vi "MM with MFC Challenge.vi"(8 "error in":errorcluster, 11 "objects IN":T1) -> (0 "error out":errorcluster, 3 "objects OUT":T1)   [LabVIEW 2011]
uses:
  Controls/Class Objects.ctl
  Modules/File/Configuration/Configuration.lvclass
  Modules/Hardware/PID/PID.lvclass
  Modules/Hardware/Power Supply/Power Supply.lvclass
  Modules/Hardware/Mass Flow Controller/Mass Flow Controller.lvclass
  Modules/Hardware/Valve Controller/Valve Controller.lvclass
  Modules/Hardware/Multimeter/Multimeter.lvclass
  Modules/Hardware/Vapour Generator/Vapour Generator.lvclass
  Modules/File/TDMS/TDMS.lvclass
  Controls/User Interface Action.ctl
  Functional Global Data/Device Params Global.ctl
  Modules/File/TDMS/Data Type.ctl
  Controls/TDMS File Handling.ctl
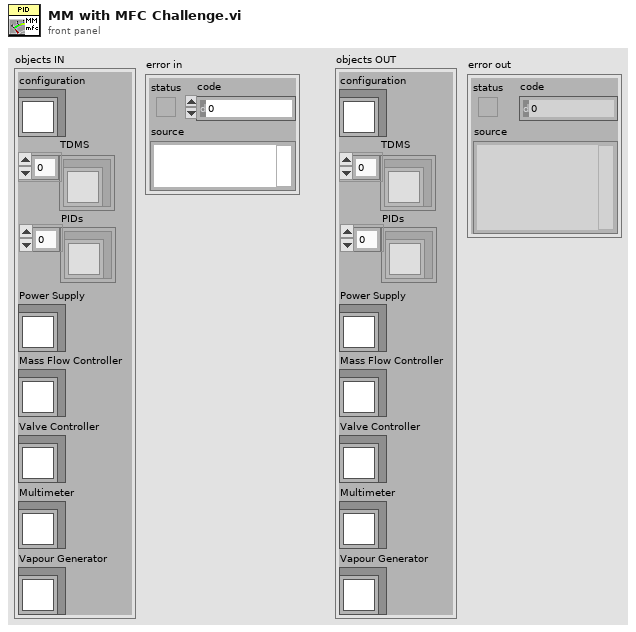
[diagram p1: front panel]
types:
  T1 = typedef "Class Objects.ctl" = cluster{"configuration":refnum<class "Configuration.lvclass">, "TDMS":refnum<class "TDMS.lvclass">[], "Power Supply":refnum<class "Power Supply.lvclass">, "Mass Flow Controller":refnum<class "Mass Flow Controller.lvclass">, "Valve Controller":refnum<class "Valve Controller.lvclass">, "Multimeter":refnum<class "Multimeter.lvclass">, "Vapour Generator":refnum<class "Vapour Generator.lvclass">, "PIDs":refnum<class "PID.lvclass">[]}
  T2 = typedef "User Interface Action.ctl" = enum16{"Initialize", "Data Acquisition Disable", "Data View Disable", "Sample Set", "Sample Set 2D Data", "Sample Set x0 & dx", "Sample Add", "Sample Set Cursor", "Sample Set Offset & Multiplier", "Sample Set Axis Labels", "Sample Parameters Disabled", "Sample Parameters Update", "Run Update", "Run Set Offset & Multiplier", "Run Set Axis Labels", "Run Set Cursor", "Run Set Disabled", "Run Parameters Update", "Run Parameters Disabled", "Run Number Set", "Run Number Set Range", "Run Number Set Disabled", "Sample Number Set", "Sample Number Set Range", "Notes Set Value", "Update Plot", "Set Plot Parameters", "Update Concentration Plot", "Time Set", "Clear DAQ Display", "Clear Analysis Display", "Status Bar Set", "Progress Bar Set", "Display Mode Set", "Experiment Type Set", "Analysis Plot Average Set", "Stop"}
  T3 = typedef "Device Params Global.ctl" = enum16{"Initialize", "Get Device Settings", "Get Device Connections", "Set Device Settings", "Set Device Connections", "Get All Device Properties"}
  T4 = typedef "TDMS.lvclass/Data Type.ctl" = enum16{"I16", "Double", "Waveform"}
  T5 = typedef "TDMS File Handling.ctl" = enum16{"Add TDMS File", "Get Active TDMS File", "Set Active TDMS File", "Set Active TDMS File Index"}
  T6 = typedef "Device Settings.ctl" = cluster{"PID":cluster{"B-M PID":T7, "INL PID":T8}, "Power Supply":cluster{"Source Value":dbl, "Source Value Units":T9, "Source Mode":T10, "Limits":T11, "Output":bool}, "Mass Flow Controller":cluster{"MFC Flow Rate":dbl, "MFC Valve Status":T14}, "Valve Controller":cluster{"Valve Assembly":T15}, "Multimeter":cluster{"Agilent 3458A":cluster{"Measurement Configuration":T17, "Measurement Integration":T18}}, "Vapour Generator":cluster{"Owlstone Permeation Tube":T19, "Owlstone GEN-SYS Setpoints":T21}}
  T7 = typedef "Baseline Mocon piD-Tech plus.lvclass/Settings.ctl" = cluster{"Detector Sampling Frequency":dbl}
  T8 = typedef "INL PID.lvclass/Settings.ctl" = cluster{"Sampling Frequency":dbl, "Integration Time":dbl, "Integration Periods":u8, "Grid Voltage":dbl}
  T9 = typedef "Power Supply.lvclass/Source Units.ctl" = enum16{"volts", "millivolts", "microvolts", "amps", "milliamps", "microamps", "nanoamps"}
  T10 = typedef "Power Supply.lvclass/Source Mode.ctl" = enum16{"Volts", "Current"}
  T11 = typedef "Power Supply.lvclass/Protection Limits.ctl" = cluster{"Voltage Limit":dbl, "Voltage Limit Units":T12, "Current Limit":dbl, "Current Limit Units":T13, "Voltage Trip/Cmpl":dbl, "Voltage Trip/Cmpl Units":T12, "Current Trip/Cmpl":dbl, "Current Trip/Cmpl Units":T13}
  T12 = typedef "Power Supply.lvclass/Voltage Units.ctl" = enum16{"volts", "millivolts", "microvolts"}
  T13 = typedef "Power Supply.lvclass/Current Units.ctl" = enum16{"amps", "milliamps", "microamps", "nanoamps"}
  T14 = typedef "Mass Flow Controller.lvclass/Valve Status.ctl" = enum16{"Open", "Closed"}
  T15 = typedef "Valve Controller.lvclass/Valve Assembly.ctl" = cluster{"Valve 1":T16, "Valve 2":T16, "Valve 3":T16, "Valve 4":T16, "Valve 5":T16}
  T16 = typedef "Valve Controller.lvclass/Status.ctl" = u16
  T17 = typedef "Agilent 3458A.lvclass/Measurement Configuration.ctl" = cluster{"Function":enum16{"DC Voltage", "AC Voltage", "AC + DC Voltage", "DC Current", "AC Current", "AC + DC Current", "2-Wire Resistance", "4-Wire Resistance", "Frequency", "Period", "Direct Sampling DC", "Direct Sampling AC", "Sub-Sampling DC", "Sub-Sampling AC"}, " Manual Resolution":enum16{"4.5", "5.5", "6.5", "7.5", "8.5"}, "Frequency Source":enum16{"AC + DC Current", "AC + DC Voltage", "AC Current", "AC Voltage"}, "Auto Range":enum16{"OFF", "ON", "ONCE"}}
  T18 = typedef "Agilent 3458A.lvclass/Measurement Integration.ctl" = cluster{"Power Line Cycles":dbl}
  T19 = typedef "Owlstone GEN-SYS.lvclass/Permeation Tube.ctl" = cluster{"Tube":T20, "Molecular Weight":dbl, "Calibration Temperature\n(Celcius)":i32, "Permeation Rate \n(ng/min)":i32}
  T20 = typedef "Owlstone GEN-SYS.lvclass/Permeation Tube Gas.ctl" = enum16{"Isobutylene 27 Nov 2012", "Ammonia 29 Sep 2012", "DMMP Tube A 3 July 2014", "DMMP Tube B 3 July 2014"}
  T21 = typedef "Owlstone GEN-SYS.lvclass/Gen-Sys Setpoints.ctl" = cluster{"OVG-4":cluster{"Oven Temperature":i32, "Sample Flow Rate":i32, "Split Flow Status":u16, "Split Flow Rate":i32}, "OHG-4":cluster{"Wet Air Flow":i32}}
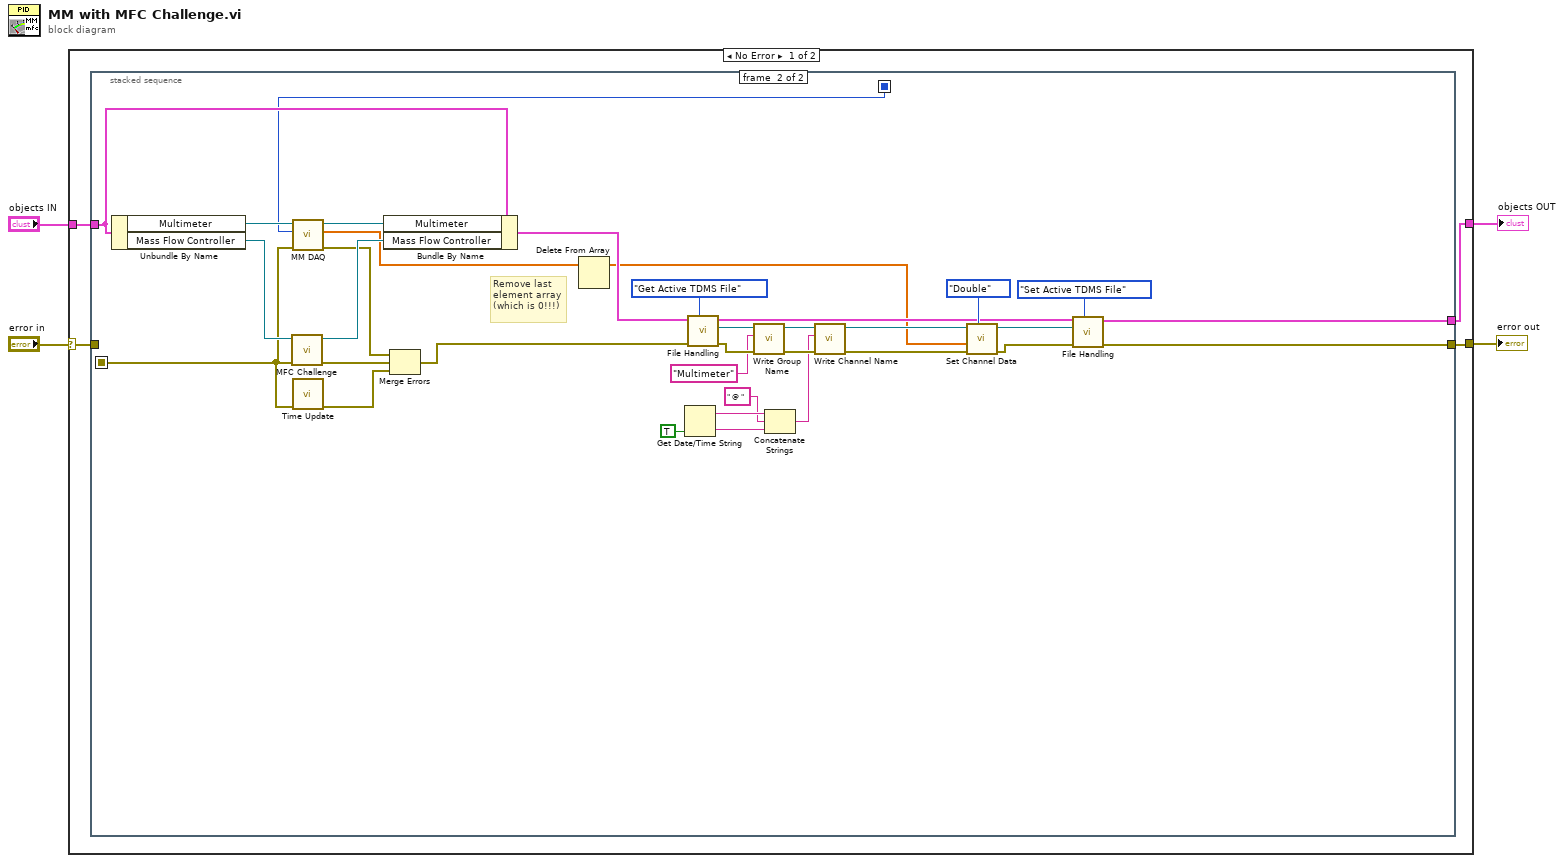
[diagram p0: block diagram]
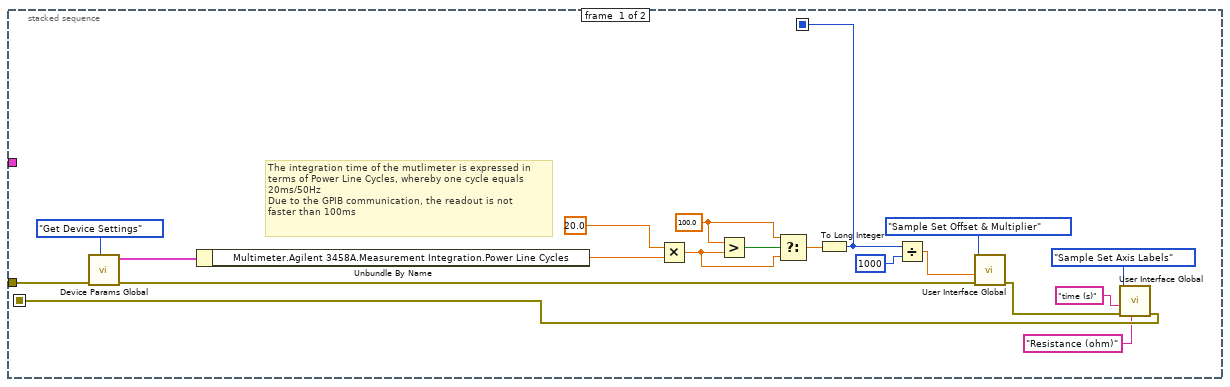
[diagram p2: hidden frame]
diagram:
  n1 = case shown="No Error" "error in" {
    selector: "error in" -> [w5 w62]
    tunnel: "objects IN" -> [w8 w63]
    tunnel: [w6 w63] -> w3
    tunnel: [w7 w62] -> w1
    frame No Error {
      n2 = stacked-sequence {
        seq-local: [w16 _] -> [_ w36]
        seq-local: [w10 _] -> [_ w29]
        tunnel: w8 -> [_ w61]
        tunnel: [_ w30] -> w7
        tunnel: [_ w53] -> w6
        tunnel: w5 -> [w25 _]
        frame #0 {
          w21 = 100.0 ("x")
          # "The integration time of the mutlimeter is expressed in\nterms of Power Line Cycles, whereby one cycle equals\n20ms/50Hz\nDue to the GPIB communication, the readout is not\nfaster than 100ms"
          n3 = call "Device Params Global.vi"("action"=Device_Params_Global."Get Device Settings", "error in"=w25) -> ("error out"=w17:errorcluster, "Device Settings OUT"=w26:T6)  [unwired: 7 in, 1 out]
          n4 = Unbundle By Name(w26) -> ("Multimeter.Agilent 3458A.Measurement Integration.Power Line Cycles"=w24:dbl)
          n5 = Multiply(x=20.0, y=w24) -> (x*y=w20:dbl)
          n6 = Greater?(x=w21, y=w20) -> (0:w22:bool)
          n7 = Select(t=w21, s=w22, f=w20) -> (s? t:f=w19:dbl)
          n8 = To Long Integer(number=w19) -> (32bit integer=w16:i32)
          n9 = Divide(x=w16, y=1000) -> (x/y=w14:dbl)
          n10 = call "User Interface Global.vi"("error in"=w17, "data1"=w14, "action"=User_Interface_Action."Sample Set Offset & Multiplier") -> ("error out"=w12:errorcluster)  [unwired: 8 in]
          n11 = call "User Interface Global.vi"("data2"="Resistance (ohm)", "error in"=w12, "data1"="time (s)", "action"=User_Interface_Action."Sample Set Axis Labels") -> ("error out"=w10:errorcluster)  [unwired: 7 in]
        }
        frame #1 {
          # "Remove last\nelement array\n(which is 0!!!)"
          n12 = Unbundle By Name(w61) -> ("Multimeter"=w38:refnum<class "Multimeter.lvclass">, "Mass Flow Controller"=w40:refnum<class "Mass Flow Controller.lvclass">)
          n13 = call "MFC Challenge.vi"("error in"=w29, "Mass Flow Controller in"=w40) -> ("error out"=w34:errorcluster, "Mass Flow Controller out"=w39:refnum<class "Mass Flow Controller.lvclass">)  [unwired: 8 in]
          n14 = call "MM DAQ.vi"("error in"=w29, "DAQ dt"=w36, "Multimeter in"=w38) -> ("error out"=w35:errorcluster, "Data"=w32:dbl[], "Multimeter out"=w37:refnum<class "Multimeter.lvclass">)  [unwired: 6 in]
          n15 = call "Time Update.vi"("error in"=w29) -> ("error out"=w28:errorcluster)  [unwired: 10 in]
          n16 = Bundle By Name(cluster=w61, "Multimeter"=w37, "Mass Flow Controller"=w39) -> (w59:T1)
          n17 = Merge Errors(w35, w34, w28) -> (w33:errorcluster)
          n18 = Delete From Array(array=w32) -> (array with subset deleted=w31:dbl[])  [unwired: 2 in, 1 out]
          n19 = Get Date/Time String(want seconds? (F)=TRUE) -> (date string=w49:string, time string=w44:string)  [unwired: 2 in]
          n20 = call "File Handling.vi"("TDMS File Handling"=TDMS_File_Handling."Get Active TDMS File", "error in"=w33, "Class objects"=w59) -> ("error out"=w51:errorcluster, "TDMS File"=w52:refnum<class "TDMS.lvclass">, "Class objects"=w54:T1)  [unwired: 6 in]
          n21 = call-dynamic "Write Group Name.vi"("error in (no error)"=w51, "Group Name"="Multimeter", "TDMS in"=w52) -> ("error out"=w47:errorcluster, "TDMS out"=w48:refnum<class "TDMS.lvclass">)  [unwired: 7 in]
          n22 = Concatenate Strings(w49, " @ " ("string"), w44) -> (w42:string)
          n23 = call-dynamic "Write Channel Name.vi"("error in (no error)"=w47, "Channel Name"=w42, "TDMS in"=w48) -> ("error out"=w46:errorcluster, "TDMS out"=w45:refnum<class "TDMS.lvclass">)  [unwired: 7 in]
          n24 = call-dynamic "Set Channel Data.vi"("data type"=Data_Type."Double", "error in"=w46, "double channel data"=w31, "TDMS in"=w45) -> ("error out"=w55:errorcluster, "TDMS out"=w57:refnum<class "TDMS.lvclass">)  [unwired: 6 in]
          n25 = call "File Handling.vi"("TDMS File Handling"=TDMS_File_Handling."Set Active TDMS File", "error in"=w55, "TDMS File"=w57, "Class objects"=w54) -> ("error out"=w30:errorcluster, "Class objects"=w53:T1)  [unwired: 5 in, 1 out]
        }
      }
    }
    frame Error {
    }
  }
  "objects OUT" <- w3
  "error out" <- w1
